vi "Choose_nest.vi"(1 "Nest":u16(ring) items=["Nest 0", "Nest 1", "Nest 2", "Nest 3", "Nest 4", "Nest 5"]) -> (0 "error out":errorcluster)   [LabVIEW 2023]
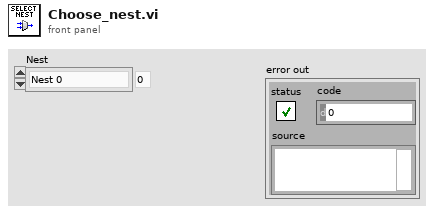
[diagram p1: front panel]
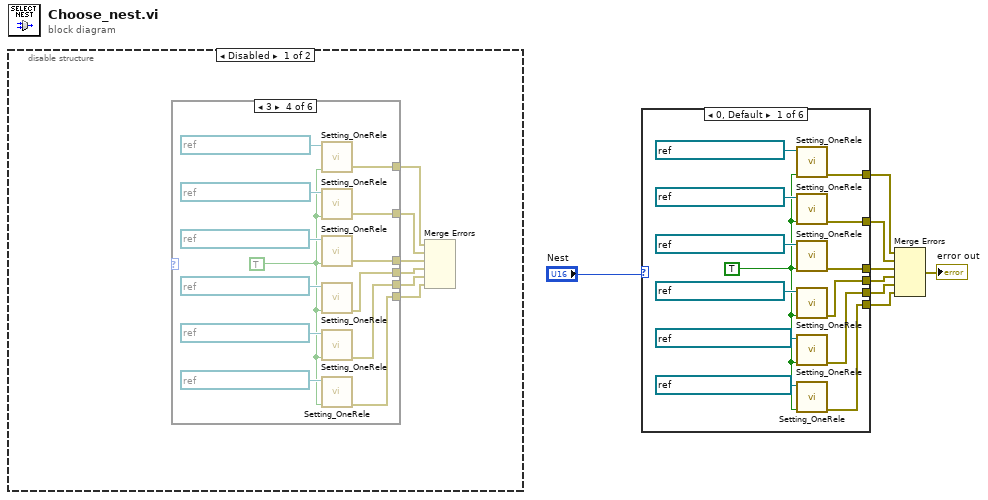
[diagram p0: block diagram]
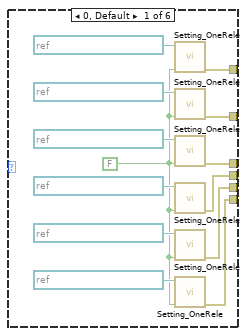
[diagram p2: hidden frame]
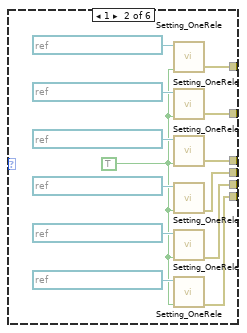
[diagram p3: hidden frame]
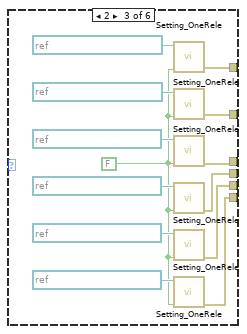
[diagram p4: hidden frame]
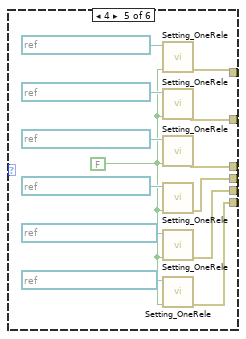
[diagram p5: hidden frame]
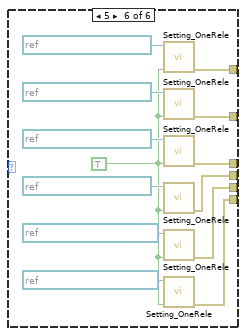
[diagram p6: hidden frame]
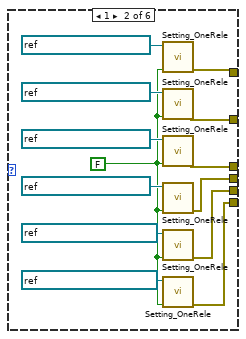
[diagram p8: hidden frame]
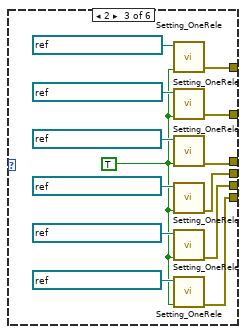
[diagram p9: hidden frame]
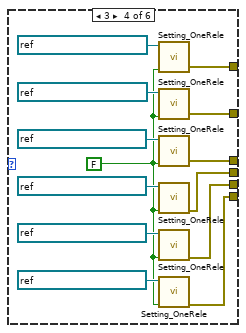
[diagram p10: hidden frame]
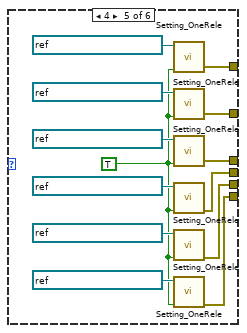
[diagram p11: hidden frame]
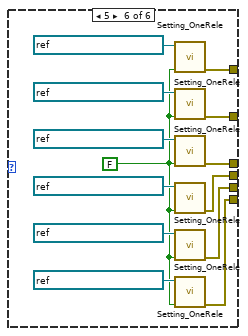
[diagram p12: hidden frame]
diagram:
  n1 = disable-structure shown="Disabled" {
    frame Disabled {
      n2 = case shown="3" {
        selector: _ -> [_ _ _ _ _ _]
        tunnel: [w21 w33 w46 w59 w72 w80] -> w14
        tunnel: [w20 w32 w45 w58 w71 w81] -> w13
        tunnel: [w19 w31 w41 w57 w70 w82] -> w12
        tunnel: [w18 w30 w42 w54 w67 w83] -> w11
        tunnel: [w17 w29 w43 w55 w68 w84] -> w10
        tunnel: [w16 w28 w44 w56 w69 w85] -> w9
        frame 0, Default {
          w15 = FALSE
          n3 = call "Setting_OneRele.vi"("data"=w15, "line"=refnum<k21> "Dev0/1stPortA/Do0") -> ("error out"=w21:errorcluster)  [unwired: 9 in]
          n4 = call "Setting_OneRele.vi"("data"=w15, "line"=refnum<k21> "Dev0/1stPortA/Do1") -> ("error out"=w20:errorcluster)  [unwired: 9 in]
          n5 = call "Setting_OneRele.vi"("data"=w15, "line"=refnum<k21> "Dev0/1stPortA/Do2") -> ("error out"=w19:errorcluster)  [unwired: 9 in]
          n6 = call "Setting_OneRele.vi"("data"=w15, "line"=refnum<k21> "Dev0/1stPortA/Do3") -> ("error out"=w18:errorcluster)  [unwired: 9 in]
          n7 = call "Setting_OneRele.vi"("data"=w15, "line"=refnum<k21> "Dev0/1stPortA/Do4") -> ("error out"=w17:errorcluster)  [unwired: 9 in]
          n8 = call "Setting_OneRele.vi"("data"=w15, "line"=refnum<k21> "Dev0/1stPortA/Do5") -> ("error out"=w16:errorcluster)  [unwired: 9 in]
        }
        frame 1 {
          w34 = TRUE
          n9 = call "Setting_OneRele.vi"("data"=w34, "line"=refnum<k21> "Dev0/1stPortA/Do0") -> ("error out"=w33:errorcluster)  [unwired: 9 in]
          n10 = call "Setting_OneRele.vi"("data"=w34, "line"=refnum<k21> "Dev0/1stPortA/Do1") -> ("error out"=w32:errorcluster)  [unwired: 9 in]
          n11 = call "Setting_OneRele.vi"("data"=w34, "line"=refnum<k21> "Dev0/1stPortA/Do2") -> ("error out"=w31:errorcluster)  [unwired: 9 in]
          n12 = call "Setting_OneRele.vi"("data"=w34, "line"=refnum<k21> "Dev0/1stPortA/Do3") -> ("error out"=w30:errorcluster)  [unwired: 9 in]
          n13 = call "Setting_OneRele.vi"("data"=w34, "line"=refnum<k21> "Dev0/1stPortA/Do4") -> ("error out"=w29:errorcluster)  [unwired: 9 in]
          n14 = call "Setting_OneRele.vi"("data"=w34, "line"=refnum<k21> "Dev0/1stPortA/Do5") -> ("error out"=w28:errorcluster)  [unwired: 9 in]
        }
        frame 2 {
          w47 = FALSE
          n15 = call "Setting_OneRele.vi"("data"=w47, "line"=refnum<k21> "Dev0/1stPortA/Do6") -> ("error out"=w46:errorcluster)  [unwired: 9 in]
          n16 = call "Setting_OneRele.vi"("data"=w47, "line"=refnum<k21> "Dev0/1stPortA/Do7") -> ("error out"=w45:errorcluster)  [unwired: 9 in]
          n17 = call "Setting_OneRele.vi"("data"=w47, "line"=refnum<k21> "Dev0/1stPortB/Do0") -> ("error out"=w41:errorcluster)  [unwired: 9 in]
          n18 = call "Setting_OneRele.vi"("data"=w47, "line"=refnum<k21> "Dev0/1stPortB/Do1") -> ("error out"=w42:errorcluster)  [unwired: 9 in]
          n19 = call "Setting_OneRele.vi"("data"=w47, "line"=refnum<k21> "Dev0/1stPortB/Do2") -> ("error out"=w43:errorcluster)  [unwired: 9 in]
          n20 = call "Setting_OneRele.vi"("data"=w47, "line"=refnum<k21> "Dev0/1stPortB/Do3") -> ("error out"=w44:errorcluster)  [unwired: 9 in]
        }
        frame 3 {
          w60 = TRUE
          n21 = call "Setting_OneRele.vi"("data"=w60, "line"=refnum<k21> "Dev0/1stPortA/Do6") -> ("error out"=w59:errorcluster)  [unwired: 9 in]
          n22 = call "Setting_OneRele.vi"("data"=w60, "line"=refnum<k21> "Dev0/1stPortA/Do7") -> ("error out"=w58:errorcluster)  [unwired: 9 in]
          n23 = call "Setting_OneRele.vi"("data"=w60, "line"=refnum<k21> "Dev0/1stPortB/Do0") -> ("error out"=w57:errorcluster)  [unwired: 9 in]
          n24 = call "Setting_OneRele.vi"("data"=w60, "line"=refnum<k21> "Dev0/1stPortB/Do1") -> ("error out"=w54:errorcluster)  [unwired: 9 in]
          n25 = call "Setting_OneRele.vi"("data"=w60, "line"=refnum<k21> "Dev0/1stPortB/Do2") -> ("error out"=w55:errorcluster)  [unwired: 9 in]
          n26 = call "Setting_OneRele.vi"("data"=w60, "line"=refnum<k21> "Dev0/1stPortB/Do3") -> ("error out"=w56:errorcluster)  [unwired: 9 in]
        }
        frame 4 {
          w73 = FALSE
          n27 = call "Setting_OneRele.vi"("data"=w73, "line"=refnum<k21> "Dev0/1stPortB/Do4") -> ("error out"=w72:errorcluster)  [unwired: 9 in]
          n28 = call "Setting_OneRele.vi"("data"=w73, "line"=refnum<k21> "Dev0/1stPortB/Do5") -> ("error out"=w71:errorcluster)  [unwired: 9 in]
          n29 = call "Setting_OneRele.vi"("data"=w73, "line"=refnum<k21> "Dev0/1stPortB/Do6") -> ("error out"=w70:errorcluster)  [unwired: 9 in]
          n30 = call "Setting_OneRele.vi"("data"=w73, "line"=refnum<k21> "Dev0/1stPortB/Do7") -> ("error out"=w67:errorcluster)  [unwired: 9 in]
          n31 = call "Setting_OneRele.vi"("data"=w73, "line"=refnum<k21> "Dev0/1stPortCL/Do0") -> ("error out"=w68:errorcluster)  [unwired: 9 in]
          n32 = call "Setting_OneRele.vi"("data"=w73, "line"=refnum<k21> "Dev0/1stPortCL/Do1") -> ("error out"=w69:errorcluster)  [unwired: 9 in]
        }
        frame 5 {
          w86 = TRUE
          n33 = call "Setting_OneRele.vi"("data"=w86, "line"=refnum<k21> "Dev0/1stPortB/Do4") -> ("error out"=w80:errorcluster)  [unwired: 9 in]
          n34 = call "Setting_OneRele.vi"("data"=w86, "line"=refnum<k21> "Dev0/1stPortB/Do5") -> ("error out"=w81:errorcluster)  [unwired: 9 in]
          n35 = call "Setting_OneRele.vi"("data"=w86, "line"=refnum<k21> "Dev0/1stPortB/Do6") -> ("error out"=w82:errorcluster)  [unwired: 9 in]
          n36 = call "Setting_OneRele.vi"("data"=w86, "line"=refnum<k21> "Dev0/1stPortB/Do7") -> ("error out"=w83:errorcluster)  [unwired: 9 in]
          n37 = call "Setting_OneRele.vi"("data"=w86, "line"=refnum<k21> "Dev0/1stPortCL/Do0") -> ("error out"=w84:errorcluster)  [unwired: 9 in]
          n38 = call "Setting_OneRele.vi"("data"=w86, "line"=refnum<k21> "Dev0/1stPortCL/Do1") -> ("error out"=w85:errorcluster)  [unwired: 9 in]
        }
      }
      n39 = Merge Errors(w14, w13, w12, w11, w10, w9) -> ()  [unwired: 1 out]
    }
    frame Enabled {
    }
  }
  n40 = case shown="0, Default" "Nest" {
    tunnel: [w93 w111 w124 w137 w150 w164] -> w8
    tunnel: [w94 w110 w123 w136 w149 w163] -> w7
    tunnel: [w95 w109 w119 w135 w148 w162] -> w6
    tunnel: [w96 w106 w120 w132 w147 w161] -> w5
    tunnel: [w97 w107 w121 w133 w146 w160] -> w4
    tunnel: [w98 w108 w122 w134 w145 w159] -> w3
    frame 0, Default {
      w99 = TRUE
      n41 = call "Setting_OneRele.vi"("data"=w99, "line"=refnum<k21> "Dev0/1stPortB/Do4") -> ("error out"=w93:errorcluster)  [unwired: 9 in]
      n42 = call "Setting_OneRele.vi"("data"=w99, "line"=refnum<k21> "Dev0/1stPortB/Do5") -> ("error out"=w94:errorcluster)  [unwired: 9 in]
      n43 = call "Setting_OneRele.vi"("data"=w99, "line"=refnum<k21> "Dev0/1stPortB/Do6") -> ("error out"=w95:errorcluster)  [unwired: 9 in]
      n44 = call "Setting_OneRele.vi"("data"=w99, "line"=refnum<k21> "Dev0/1stPortB/Do7") -> ("error out"=w96:errorcluster)  [unwired: 9 in]
      n45 = call "Setting_OneRele.vi"("data"=w99, "line"=refnum<k21> "Dev0/1stPortCL/Do0") -> ("error out"=w97:errorcluster)  [unwired: 9 in]
      n46 = call "Setting_OneRele.vi"("data"=w99, "line"=refnum<k21> "Dev0/1stPortCL/Do1") -> ("error out"=w98:errorcluster)  [unwired: 9 in]
    }
    frame 1 {
      w112 = FALSE
      n47 = call "Setting_OneRele.vi"("data"=w112, "line"=refnum<k21> "Dev0/1stPortB/Do4") -> ("error out"=w111:errorcluster)  [unwired: 9 in]
      n48 = call "Setting_OneRele.vi"("data"=w112, "line"=refnum<k21> "Dev0/1stPortB/Do5") -> ("error out"=w110:errorcluster)  [unwired: 9 in]
      n49 = call "Setting_OneRele.vi"("data"=w112, "line"=refnum<k21> "Dev0/1stPortB/Do6") -> ("error out"=w109:errorcluster)  [unwired: 9 in]
      n50 = call "Setting_OneRele.vi"("data"=w112, "line"=refnum<k21> "Dev0/1stPortB/Do7") -> ("error out"=w106:errorcluster)  [unwired: 9 in]
      n51 = call "Setting_OneRele.vi"("data"=w112, "line"=refnum<k21> "Dev0/1stPortCL/Do0") -> ("error out"=w107:errorcluster)  [unwired: 9 in]
      n52 = call "Setting_OneRele.vi"("data"=w112, "line"=refnum<k21> "Dev0/1stPortCL/Do1") -> ("error out"=w108:errorcluster)  [unwired: 9 in]
    }
    frame 2 {
      w125 = TRUE
      n53 = call "Setting_OneRele.vi"("data"=w125, "line"=refnum<k21> "Dev0/1stPortA/Do6") -> ("error out"=w124:errorcluster)  [unwired: 9 in]
      n54 = call "Setting_OneRele.vi"("data"=w125, "line"=refnum<k21> "Dev0/1stPortA/Do7") -> ("error out"=w123:errorcluster)  [unwired: 9 in]
      n55 = call "Setting_OneRele.vi"("data"=w125, "line"=refnum<k21> "Dev0/1stPortB/Do0") -> ("error out"=w119:errorcluster)  [unwired: 9 in]
      n56 = call "Setting_OneRele.vi"("data"=w125, "line"=refnum<k21> "Dev0/1stPortB/Do1") -> ("error out"=w120:errorcluster)  [unwired: 9 in]
      n57 = call "Setting_OneRele.vi"("data"=w125, "line"=refnum<k21> "Dev0/1stPortB/Do2") -> ("error out"=w121:errorcluster)  [unwired: 9 in]
      n58 = call "Setting_OneRele.vi"("data"=w125, "line"=refnum<k21> "Dev0/1stPortB/Do3") -> ("error out"=w122:errorcluster)  [unwired: 9 in]
    }
    frame 3 {
      w138 = FALSE
      n59 = call "Setting_OneRele.vi"("data"=w138, "line"=refnum<k21> "Dev0/1stPortA/Do6") -> ("error out"=w137:errorcluster)  [unwired: 9 in]
      n60 = call "Setting_OneRele.vi"("data"=w138, "line"=refnum<k21> "Dev0/1stPortA/Do7") -> ("error out"=w136:errorcluster)  [unwired: 9 in]
      n61 = call "Setting_OneRele.vi"("data"=w138, "line"=refnum<k21> "Dev0/1stPortB/Do0") -> ("error out"=w135:errorcluster)  [unwired: 9 in]
      n62 = call "Setting_OneRele.vi"("data"=w138, "line"=refnum<k21> "Dev0/1stPortB/Do1") -> ("error out"=w132:errorcluster)  [unwired: 9 in]
      n63 = call "Setting_OneRele.vi"("data"=w138, "line"=refnum<k21> "Dev0/1stPortB/Do2") -> ("error out"=w133:errorcluster)  [unwired: 9 in]
      n64 = call "Setting_OneRele.vi"("data"=w138, "line"=refnum<k21> "Dev0/1stPortB/Do3") -> ("error out"=w134:errorcluster)  [unwired: 9 in]
    }
    frame 4 {
      w151 = TRUE
      n65 = call "Setting_OneRele.vi"("data"=w151, "line"=refnum<k21> "Dev0/1stPortA/Do0") -> ("error out"=w150:errorcluster)  [unwired: 9 in]
      n66 = call "Setting_OneRele.vi"("data"=w151, "line"=refnum<k21> "Dev0/1stPortA/Do1") -> ("error out"=w149:errorcluster)  [unwired: 9 in]
      n67 = call "Setting_OneRele.vi"("data"=w151, "line"=refnum<k21> "Dev0/1stPortA/Do2") -> ("error out"=w148:errorcluster)  [unwired: 9 in]
      n68 = call "Setting_OneRele.vi"("data"=w151, "line"=refnum<k21> "Dev0/1stPortA/Do3") -> ("error out"=w147:errorcluster)  [unwired: 9 in]
      n69 = call "Setting_OneRele.vi"("data"=w151, "line"=refnum<k21> "Dev0/1stPortA/Do4") -> ("error out"=w146:errorcluster)  [unwired: 9 in]
      n70 = call "Setting_OneRele.vi"("data"=w151, "line"=refnum<k21> "Dev0/1stPortA/Do5") -> ("error out"=w145:errorcluster)  [unwired: 9 in]
    }
    frame 5 {
      w158 = FALSE
      n71 = call "Setting_OneRele.vi"("data"=w158, "line"=refnum<k21> "Dev0/1stPortA/Do0") -> ("error out"=w164:errorcluster)  [unwired: 9 in]
      n72 = call "Setting_OneRele.vi"("data"=w158, "line"=refnum<k21> "Dev0/1stPortA/Do1") -> ("error out"=w163:errorcluster)  [unwired: 9 in]
      n73 = call "Setting_OneRele.vi"("data"=w158, "line"=refnum<k21> "Dev0/1stPortA/Do2") -> ("error out"=w162:errorcluster)  [unwired: 9 in]
      n74 = call "Setting_OneRele.vi"("data"=w158, "line"=refnum<k21> "Dev0/1stPortA/Do3") -> ("error out"=w161:errorcluster)  [unwired: 9 in]
      n75 = call "Setting_OneRele.vi"("data"=w158, "line"=refnum<k21> "Dev0/1stPortA/Do4") -> ("error out"=w160:errorcluster)  [unwired: 9 in]
      n76 = call "Setting_OneRele.vi"("data"=w158, "line"=refnum<k21> "Dev0/1stPortA/Do5") -> ("error out"=w159:errorcluster)  [unwired: 9 in]
    }
  }
  n77 = Merge Errors(w8, w7, w6, w5, w4, w3) -> (→"error out":errorcluster)
